vi "RunMeas.vi"(8 "error in (no error)":errorcluster, 11 "NhRegenGridSim in":refnum<class "NHRGridSim.lvclass">) -> (0 "error out":errorcluster, 2 "variant":variant, 3 "NhRegenGridSim out":refnum<class "NHRGridSim.lvclass">)   [LabVIEW 2018, in "AcPwrPlugins.lvlib" / "NHRGridSim.lvclass"]
doc: "This VI acquires data from the instrument and fetches the data from instrument memory into LabVIEW memory."
uses:
  NHRGridSim.lvclass
  C:/Users/ico/Documents/Projects/NistPluggableModules/AcPwr/AcPwrPlugins/AcPwrBaseClass/AcPwrBase.lvclass
  <instrlib>/NH Research 9400 Series/Public/Data/Low Level/Fetch (Ave Current).vi
  <instrlib>/NH Research 9400 Series/Public/Data/Read (Ave Current).vi
  <instrlib>/NH Research 9400 Series/Public/Data/Low Level/Fetch (Max Current).vi
  <instrlib>/NH Research 9400 Series/Public/Data/Read (Max Current).vi
  <instrlib>/NH Research 9400 Series/Public/Data/Low Level/Fetch (Min Current).vi
  <instrlib>/NH Research 9400 Series/Public/Data/Read (Min Current).vi
  <instrlib>/NH Research 9400 Series/Public/Data/Low Level/Fetch (Ave Voltage).vi
  <instrlib>/NH Research 9400 Series/Public/Data/Read (Ave Voltage).vi
  <instrlib>/NH Research 9400 Series/Public/Data/Low Level/Fetch (Max Voltage).vi
  <instrlib>/NH Research 9400 Series/Public/Data/Read (Max Voltage).vi
  <instrlib>/NH Research 9400 Series/Public/Data/Low Level/Fetch (Min Voltage).vi
  <instrlib>/NH Research 9400 Series/Public/Data/Read (Min Voltage).vi
  <instrlib>/NH Research 9400 Series/Public/Data/Low Level/Fetch (Ave True Power).vi
  <instrlib>/NH Research 9400 Series/Public/Data/Read (Ave True Power).vi
  <instrlib>/NH Research 9400 Series/Public/Data/Low Level/Fetch (Max True Power).vi
  <instrlib>/NH Research 9400 Series/Public/Data/Read (Max True Power).vi
  <instrlib>/NH Research 9400 Series/Public/Data/Low Level/Fetch (Min True Power).vi
  <instrlib>/NH Research 9400 Series/Public/Data/Read (Min True Power).vi
  <instrlib>/NH Research 9400 Series/Public/Data/Low Level/Fetch (Ave Apparent Power).vi
  <instrlib>/NH Research 9400 Series/Public/Data/Read (Ave Apparent Power).vi
  <instrlib>/NH Research 9400 Series/Public/Data/Low Level/Fetch (Max Apparent Power).vi
  <instrlib>/NH Research 9400 Series/Public/Data/Read (Max Apparent Power).vi
  <instrlib>/NH Research 9400 Series/Public/Data/Low Level/Fetch (Min Apparent Power).vi
  <instrlib>/NH Research 9400 Series/Public/Data/Read (Min Apparent Power).vi
  <instrlib>/NH Research 9400 Series/Public/Data/Low Level/Fetch (Power Factor).vi
  <instrlib>/NH Research 9400 Series/Public/Data/Read (Power Factor).vi
  <instrlib>/NH Research 9400 Series/Public/Data/Low Level/Fetch (Crest Factor).vi
  <instrlib>/NH Research 9400 Series/Public/Data/Read (Crest Factor).vi
  <instrlib>/NH Research 9400 Series/NH Research 9400 Series.lvlib
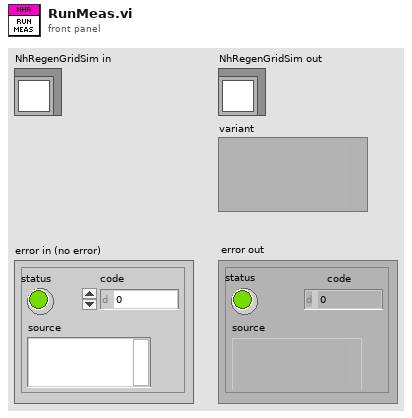
[diagram p1: front panel]
types:
  T1 = typedef "AcPwrPlugins.lvlib/NhRegenGridSim.lvclass/Measurements.ctl" = cluster{"Handle":string, "Name":string, "Enabled ":bool, "Measurement Value":dbl, "Measurement Type ":enum16{"Average Current", "Max Current", "Min Current", "Average Voltage", "Max Voltage", "Min Voltage", "Average True Power", "Max True Power", "Min True Power", "Average Apparent Power", "Max Apparent Power", "Min Apparent Power", "Power Factor", "Crest Factor"}, "Phase ":i32, "btnMeasFetch":bool}[]
  T2 = enum16{"Average Current", "Max Current", "Min Current", "Average Voltage", "Max Voltage", "Min Voltage", "Average True Power", "Max True Power", "Min True Power", "Average Apparent Power", "Max Apparent Power", "Min Apparent Power", "Power Factor", "Crest Factor"}
  T3 = cluster{"Handle":string, "Name":string, "Enabled ":bool, "Measurement Value":dbl, "Measurement Type ":enum16{"Average Current", "Max Current", "Min Current", "Average Voltage", "Max Voltage", "Min Voltage", "Average True Power", "Max True Power", "Min True Power", "Average Apparent Power", "Max Apparent Power", "Min Apparent Power", "Power Factor", "Crest Factor"}, "Phase ":i32, "btnMeasFetch":bool}
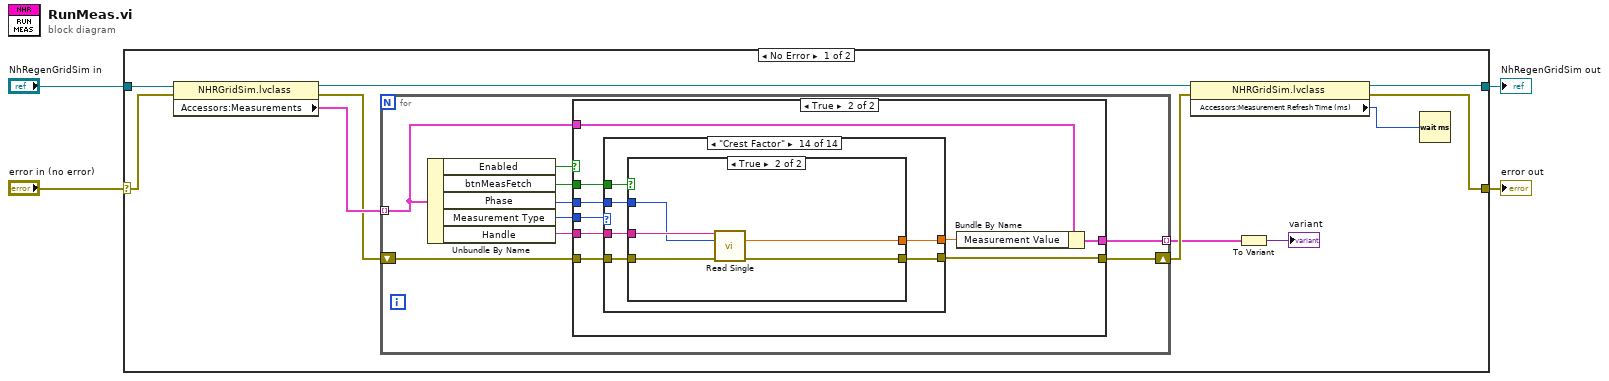
[diagram p0: block diagram]
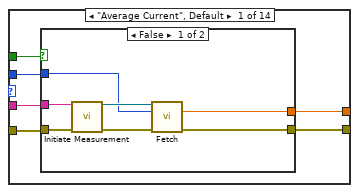
[diagram p3: hidden frame]
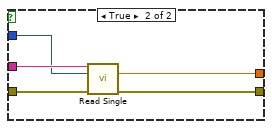
[diagram p4: hidden frame]
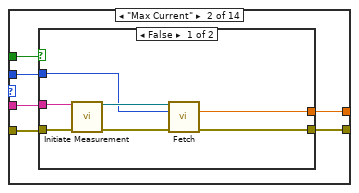
[diagram p5: hidden frame]
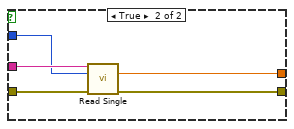
[diagram p6: hidden frame]
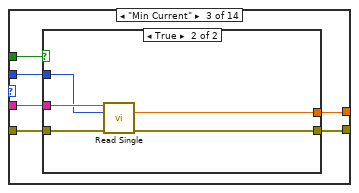
[diagram p7: hidden frame]
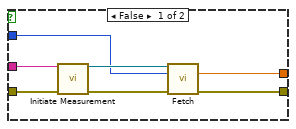
[diagram p8: hidden frame]
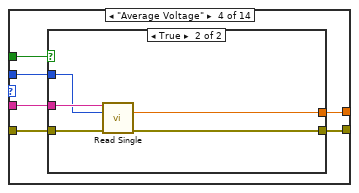
[diagram p9: hidden frame]
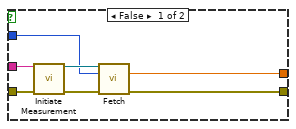
[diagram p10: hidden frame]
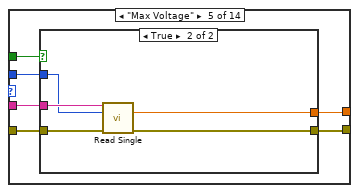
[diagram p11: hidden frame]
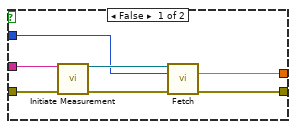
[diagram p12: hidden frame]
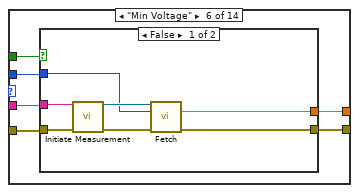
[diagram p13: hidden frame]
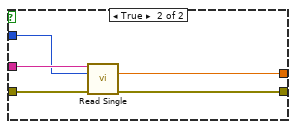
[diagram p14: hidden frame]
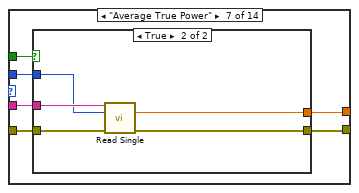
[diagram p15: hidden frame]
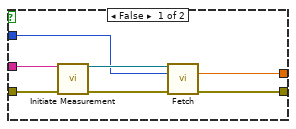
[diagram p16: hidden frame]
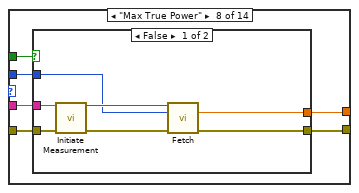
[diagram p17: hidden frame]
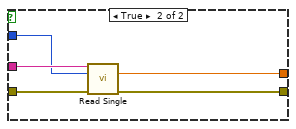
[diagram p18: hidden frame]
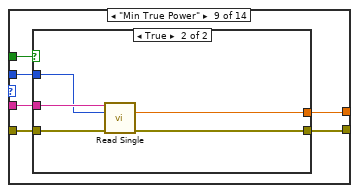
[diagram p19: hidden frame]
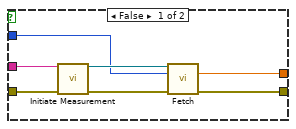
[diagram p20: hidden frame]
diagram:
  n1 = case shown="No Error" "error in (no error)" {
    selector: "error in (no error)" -> [w14 w287]
    tunnel: [w8 w287] -> w4
    tunnel: [w9 w288] -> w3
    tunnel: "NhRegenGridSim in" -> [w15 w288]
    frame No Error {
      n2 = property class="NHRGridSim.lvclass"(reference=w15, error in=w14) -> (reference out=w11:refnum<class "NHRGridSim.lvclass">, error out=w12:errorcluster, "Accessors:Measurements"=w13:T1)
      n3 = for {
        tunnel: w13 -> [w24] mode=indexing
        shift-right: [w21] -> w10
        shift-left: w12 -> [w23]
        tunnel: [w18] -> w5 mode=indexing
        n4 = Unbundle By Name(w24) -> ("Enabled"=w16:bool, "btnMeasFetch"=w20:bool, "Phase"=w19:i32, "Measurement Type"=w17:T2, "Handle"=w22:string)
        n5 = case shown="True" w16 {
          tunnel: w24 -> [_ w33]
          tunnel: w23 -> [w25 w30]
          tunnel: w22 -> [_ w29]
          tunnel: [w25 w27] -> w21
          tunnel: w19 -> [_ w31]
          tunnel: [_ w34] -> w18
          tunnel: w17 -> [_ w32]
          tunnel: w20 -> [_ w28]
          frame False {
          }
          frame True {
            n6 = case shown="\"Crest Factor\"" w32 {
              tunnel: w31 -> [w37 w54 w72 w90 w108 w126 w144 w162 w180 w198 w216 w234 w252 w270]
              tunnel: w30 -> [w40 w58 w74 w92 w110 w128 w146 w164 w182 w200 w218 w236 w254 w272]
              tunnel: w29 -> [w38 w55 w73 w91 w109 w127 w145 w163 w181 w199 w217 w235 w253 w271]
              tunnel: w28 -> [w36 w53 w71 w89 w107 w125 w143 w161 w179 w197 w215 w233 w251 w269]
              tunnel: [w39 w57 w76 w94 w112 w130 w148 w166 w184 w202 w220 w238 w256 w274] -> w27
              tunnel: [w35 w56 w75 w93 w111 w129 w147 w165 w183 w201 w219 w237 w255 w273] -> w26
              frame "Average Current", Default {
                n7 = case shown="False" w36 {
                  tunnel: w40 -> [w47 w52]
                  tunnel: w38 -> [w46 w51]
                  tunnel: [w42 w50] -> w39
                  tunnel: [w41 w49] -> w35
                  tunnel: w37 -> [w43 w48]
                  frame False {
                    n8 = call <instrlib>:"Initiate Measurement.vi"("VISA resource name"=w46, "error in (no error)"=w47) -> ("VISA resource name out"=w44:refnum<visa-resource-name>, "error out"=w45:errorcluster)  [unwired: 12 in]
                    n9 = call-poly <instrlib>:"Fetch.vi"("VISA resource name"=w44, "Phase (0: All)"=w43, "error in (no error)"=w45) -> ("Ave Current (A)"=w41:dbl, "error out"=w42:errorcluster)  [unwired: 10 in, 1 out]
                  }
                  frame True {
                    n10 = call-poly <instrlib>:"Read Single.vi"("VISA resource name"=w51, "Phase (0: All)"=w48, "error in (no error)"=w52) -> ("Ave Current (A)"=w49:dbl, "error out"=w50:errorcluster)  [unwired: 10 in, 1 out]
                  }
                }
              }
              frame "Max Current" {
                n11 = case shown="False" w53 {
                  tunnel: w58 -> [w65 w70]
                  tunnel: w55 -> [w64 w69]
                  tunnel: [w60 w68] -> w57
                  tunnel: [w59 w67] -> w56
                  tunnel: w54 -> [w61 w66]
                  frame False {
                    n12 = call <instrlib>:"Initiate Measurement.vi"("VISA resource name"=w64, "error in (no error)"=w65) -> ("VISA resource name out"=w62:refnum<visa-resource-name>, "error out"=w63:errorcluster)  [unwired: 12 in]
                    n13 = call-poly <instrlib>:"Fetch.vi"("VISA resource name"=w62, "Phase (0: All)"=w61, "error in (no error)"=w63) -> ("Max Current (A)"=w59:dbl, "error out"=w60:errorcluster)  [unwired: 10 in, 1 out]
                  }
                  frame True {
                    n14 = call-poly <instrlib>:"Read Single.vi"("VISA resource name"=w69, "Phase (0: All)"=w66, "error in (no error)"=w70) -> ("Max Current (A)"=w67:dbl, "error out"=w68:errorcluster)  [unwired: 10 in, 1 out]
                  }
                }
              }
              frame "Min Current" {
                n15 = case shown="True" w71 {
                  tunnel: w74 -> [w83 w88]
                  tunnel: w73 -> [w82 w87]
                  tunnel: [w78 w86] -> w76
                  tunnel: [w77 w85] -> w75
                  tunnel: w72 -> [w79 w84]
                  frame False {
                    n16 = call <instrlib>:"Initiate Measurement.vi"("VISA resource name"=w82, "error in (no error)"=w83) -> ("VISA resource name out"=w80:refnum<visa-resource-name>, "error out"=w81:errorcluster)  [unwired: 12 in]
                    n17 = call-poly <instrlib>:"Fetch.vi"("VISA resource name"=w80, "Phase (0: All)"=w79, "error in (no error)"=w81) -> ("Min Current (A)"=w77:dbl, "error out"=w78:errorcluster)  [unwired: 10 in, 1 out]
                  }
                  frame True {
                    n18 = call-poly <instrlib>:"Read Single.vi"("VISA resource name"=w87, "Phase (0: All)"=w84, "error in (no error)"=w88) -> ("Min Current (A)"=w85:dbl, "error out"=w86:errorcluster)  [unwired: 10 in, 1 out]
                  }
                }
              }
              frame "Average Voltage" {
                n19 = case shown="True" w89 {
                  tunnel: w92 -> [w101 w106]
                  tunnel: w91 -> [w100 w105]
                  tunnel: [w96 w104] -> w94
                  tunnel: [w95 w103] -> w93
                  tunnel: w90 -> [w97 w102]
                  frame False {
                    n20 = call <instrlib>:"Initiate Measurement.vi"("VISA resource name"=w100, "error in (no error)"=w101) -> ("VISA resource name out"=w98:refnum<visa-resource-name>, "error out"=w99:errorcluster)  [unwired: 12 in]
                    n21 = call-poly <instrlib>:"Fetch.vi"("VISA resource name"=w98, "Phase (0: All)"=w97, "error in (no error)"=w99) -> ("Ave Voltage (V)"=w95:dbl, "error out"=w96:errorcluster)  [unwired: 10 in, 1 out]
                  }
                  frame True {
                    n22 = call-poly <instrlib>:"Read Single.vi"("VISA resource name"=w105, "Phase (0: All)"=w102, "error in (no error)"=w106) -> ("Ave Voltage (V)"=w103:dbl, "error out"=w104:errorcluster)  [unwired: 10 in, 1 out]
                  }
                }
              }
              frame "Max Voltage" {
                n23 = case shown="True" w107 {
                  tunnel: w110 -> [w119 w124]
                  tunnel: w109 -> [w118 w123]
                  tunnel: [w114 w122] -> w112
                  tunnel: [w113 w121] -> w111
                  tunnel: w108 -> [w115 w120]
                  frame False {
                    n24 = call <instrlib>:"Initiate Measurement.vi"("VISA resource name"=w118, "error in (no error)"=w119) -> ("VISA resource name out"=w116:refnum<visa-resource-name>, "error out"=w117:errorcluster)  [unwired: 12 in]
                    n25 = call-poly <instrlib>:"Fetch.vi"("VISA resource name"=w116, "Phase (0: All)"=w115, "error in (no error)"=w117) -> ("Max Voltage (V)"=w113:dbl, "error out"=w114:errorcluster)  [unwired: 10 in, 1 out]
                  }
                  frame True {
                    n26 = call-poly <instrlib>:"Read Single.vi"("VISA resource name"=w123, "Phase (0: All)"=w120, "error in (no error)"=w124) -> ("Max Voltage (V)"=w121:dbl, "error out"=w122:errorcluster)  [unwired: 10 in, 1 out]
                  }
                }
              }
              frame "Min Voltage" {
                n27 = case shown="False" w125 {
                  tunnel: w128 -> [w137 w142]
                  tunnel: w127 -> [w136 w141]
                  tunnel: [w132 w140] -> w130
                  tunnel: [w131 w139] -> w129
                  tunnel: w126 -> [w133 w138]
                  frame False {
                    n28 = call <instrlib>:"Initiate Measurement.vi"("VISA resource name"=w136, "error in (no error)"=w137) -> ("VISA resource name out"=w134:refnum<visa-resource-name>, "error out"=w135:errorcluster)  [unwired: 12 in]
                    n29 = call-poly <instrlib>:"Fetch.vi"("VISA resource name"=w134, "Phase (0: All)"=w133, "error in (no error)"=w135) -> ("Min Voltage (V)"=w131:dbl, "error out"=w132:errorcluster)  [unwired: 10 in, 1 out]
                  }
                  frame True {
                    n30 = call-poly <instrlib>:"Read Single.vi"("VISA resource name"=w141, "Phase (0: All)"=w138, "error in (no error)"=w142) -> ("Min Voltage (V)"=w139:dbl, "error out"=w140:errorcluster)  [unwired: 10 in, 1 out]
                  }
                }
              }
              frame "Average True Power" {
                n31 = case shown="True" w143 {
                  tunnel: w146 -> [w155 w160]
                  tunnel: w145 -> [w154 w159]
                  tunnel: [w150 w158] -> w148
                  tunnel: [w149 w157] -> w147
                  tunnel: w144 -> [w151 w156]
                  frame False {
                    n32 = call <instrlib>:"Initiate Measurement.vi"("VISA resource name"=w154, "error in (no error)"=w155) -> ("VISA resource name out"=w152:refnum<visa-resource-name>, "error out"=w153:errorcluster)  [unwired: 12 in]
                    n33 = call-poly <instrlib>:"Fetch.vi"("VISA resource name"=w152, "Phase (0: All)"=w151, "error in (no error)"=w153) -> ("Ave True Power (W)"=w149:dbl, "error out"=w150:errorcluster)  [unwired: 10 in, 1 out]
                  }
                  frame True {
                    n34 = call-poly <instrlib>:"Read Single.vi"("VISA resource name"=w159, "Phase (0: All)"=w156, "error in (no error)"=w160) -> ("True Power (W)"=w157:dbl, "error out"=w158:errorcluster)  [unwired: 10 in, 1 out]
                  }
                }
              }
              frame "Max True Power" {
                n35 = case shown="False" w161 {
                  tunnel: w164 -> [w173 w178]
                  tunnel: w163 -> [w172 w177]
                  tunnel: [w168 w176] -> w166
                  tunnel: [w167 w175] -> w165
                  tunnel: w162 -> [w169 w174]
                  frame False {
                    n36 = call <instrlib>:"Initiate Measurement.vi"("VISA resource name"=w172, "error in (no error)"=w173) -> ("VISA resource name out"=w170:refnum<visa-resource-name>, "error out"=w171:errorcluster)  [unwired: 12 in]
                    n37 = call-poly <instrlib>:"Fetch.vi"("VISA resource name"=w170, "Phase (0: All)"=w169, "error in (no error)"=w171) -> ("Max True Power (W)"=w167:dbl, "error out"=w168:errorcluster)  [unwired: 10 in, 1 out]
                  }
                  frame True {
                    n38 = call-poly <instrlib>:"Read Single.vi"("VISA resource name"=w177, "Phase (0: All)"=w174, "error in (no error)"=w178) -> ("Max True Power (W)"=w175:dbl, "error out"=w176:errorcluster)  [unwired: 10 in, 1 out]
                  }
                }
              }
              frame "Min True Power" {
                n39 = case shown="True" w179 {
                  tunnel: w182 -> [w191 w196]
                  tunnel: w181 -> [w190 w195]
                  tunnel: [w186 w194] -> w184
                  tunnel: [w185 w193] -> w183
                  tunnel: w180 -> [w187 w192]
                  frame False {
                    n40 = call <instrlib>:"Initiate Measurement.vi"("VISA resource name"=w190, "error in (no error)"=w191) -> ("VISA resource name out"=w188:refnum<visa-resource-name>, "error out"=w189:errorcluster)  [unwired: 12 in]
                    n41 = call-poly <instrlib>:"Fetch.vi"("VISA resource name"=w188, "Phase (0: All)"=w187, "error in (no error)"=w189) -> ("Min True Power (W)"=w185:dbl, "error out"=w186:errorcluster)  [unwired: 10 in, 1 out]
                  }
                  frame True {
                    n42 = call-poly <instrlib>:"Read Single.vi"("VISA resource name"=w195, "Phase (0: All)"=w192, "error in (no error)"=w196) -> ("Min True Power (W)"=w193:dbl, "error out"=w194:errorcluster)  [unwired: 10 in, 1 out]
                  }
                }
              }
              frame "Average Apparent Power" {
                n43 = case shown="False" w197 {
                  tunnel: w200 -> [w209 w214]
                  tunnel: w199 -> [w208 w213]
                  tunnel: [w204 w212] -> w202
                  tunnel: [w203 w211] -> w201
                  tunnel: w198 -> [w205 w210]
                  frame False {
                    n44 = call <instrlib>:"Initiate Measurement.vi"("VISA resource name"=w208, "error in (no error)"=w209) -> ("VISA resource name out"=w206:refnum<visa-resource-name>, "error out"=w207:errorcluster)  [unwired: 12 in]
                    n45 = call-poly <instrlib>:"Fetch.vi"("VISA resource name"=w206, "Phase (0: All)"=w205, "error in (no error)"=w207) -> ("Apparent Power (VA)"=w203:dbl, "error out"=w204:errorcluster)  [unwired: 10 in, 1 out]
                  }
                  frame True {
                    n46 = call-poly <instrlib>:"Read Single.vi"("VISA resource name"=w213, "Phase (0: All)"=w210, "error in (no error)"=w214) -> ("Apparent Power (VA)"=w211:dbl, "error out"=w212:errorcluster)  [unwired: 10 in, 1 out]
                  }
                }
              }
              frame "Max Apparent Power" {
                n47 = case shown="True" w215 {
                  tunnel: w218 -> [w227 w232]
                  tunnel: w217 -> [w226 w231]
                  tunnel: [w222 w230] -> w220
                  tunnel: [w221 w229] -> w219
                  tunnel: w216 -> [w223 w228]
                  frame False {
                    n48 = call <instrlib>:"Initiate Measurement.vi"("VISA resource name"=w226, "error in (no error)"=w227) -> ("VISA resource name out"=w224:refnum<visa-resource-name>, "error out"=w225:errorcluster)  [unwired: 12 in]
                    n49 = call-poly <instrlib>:"Fetch.vi"("VISA resource name"=w224, "Phase (0: All)"=w223, "error in (no error)"=w225) -> ("Max Apparent Power (VA)"=w221:dbl, "error out"=w222:errorcluster)  [unwired: 10 in, 1 out]
                  }
                  frame True {
                    n50 = call-poly <instrlib>:"Read Single.vi"("VISA resource name"=w231, "Phase (0: All)"=w228, "error in (no error)"=w232) -> ("Max Apparent Power (VA)"=w229:dbl, "error out"=w230:errorcluster)  [unwired: 10 in, 1 out]
                  }
                }
              }
              frame "Min Apparent Power" {
                n51 = case shown="False" w233 {
                  tunnel: w236 -> [w245 w250]
                  tunnel: w235 -> [w244 w249]
                  tunnel: [w240 w248] -> w238
                  tunnel: [w239 w247] -> w237
                  tunnel: w234 -> [w241 w246]
                  frame False {
                    n52 = call <instrlib>:"Initiate Measurement.vi"("VISA resource name"=w244, "error in (no error)"=w245) -> ("VISA resource name out"=w242:refnum<visa-resource-name>, "error out"=w243:errorcluster)  [unwired: 12 in]
                    n53 = call-poly <instrlib>:"Fetch.vi"("VISA resource name"=w242, "Phase (0: All)"=w241, "error in (no error)"=w243) -> ("Min Apparent Power (VA)"=w239:dbl, "error out"=w240:errorcluster)  [unwired: 10 in, 1 out]
                  }
                  frame True {
                    n54 = call-poly <instrlib>:"Read Single.vi"("VISA resource name"=w249, "Phase (0: All)"=w246, "error in (no error)"=w250) -> ("Min Apparent Power (VA)"=w247:dbl, "error out"=w248:errorcluster)  [unwired: 10 in, 1 out]
                  }
                }
              }
              frame "Power Factor" {
                n55 = case shown="True" w251 {
                  tunnel: w254 -> [w263 w268]
                  tunnel: w253 -> [w262 w267]
                  tunnel: [w258 w266] -> w256
                  tunnel: [w257 w265] -> w255
                  tunnel: w252 -> [w259 w264]
                  frame False {
                    n56 = call <instrlib>:"Initiate Measurement.vi"("VISA resource name"=w262, "error in (no error)"=w263) -> ("VISA resource name out"=w260:refnum<visa-resource-name>, "error out"=w261:errorcluster)  [unwired: 12 in]
                    n57 = call-poly <instrlib>:"Fetch.vi"("VISA resource name"=w260, "Phase (0: All)"=w259, "error in (no error)"=w261) -> ("Power Factor"=w257:dbl, "error out"=w258:errorcluster)  [unwired: 10 in, 1 out]
                  }
                  frame True {
                    n58 = call-poly <instrlib>:"Read Single.vi"("VISA resource name"=w267, "Phase (0: All)"=w264, "error in (no error)"=w268) -> ("Power Factor"=w265:dbl, "error out"=w266:errorcluster)  [unwired: 10 in, 1 out]
                  }
                }
              }
              frame "Crest Factor" {
                n59 = case shown="True" w269 {
                  tunnel: w272 -> [w281 w286]
                  tunnel: w271 -> [w280 w285]
                  tunnel: [w276 w284] -> w274
                  tunnel: [w275 w283] -> w273
                  tunnel: w270 -> [w277 w282]
                  frame False {
                    n60 = call <instrlib>:"Initiate Measurement.vi"("VISA resource name"=w280, "error in (no error)"=w281) -> ("VISA resource name out"=w278:refnum<visa-resource-name>, "error out"=w279:errorcluster)  [unwired: 12 in]
                    n61 = call-poly <instrlib>:"Fetch.vi"("VISA resource name"=w278, "Phase (0: All)"=w277, "error in (no error)"=w279) -> ("Crest Factor"=w275:dbl, "error out"=w276:errorcluster)  [unwired: 10 in, 1 out]
                  }
                  frame True {
                    n62 = call-poly <instrlib>:"Read Single.vi"("VISA resource name"=w285, "Phase (0: All)"=w282, "error in (no error)"=w286) -> ("Crest Factor"=w283:dbl, "error out"=w284:errorcluster)  [unwired: 10 in, 1 out]
                  }
                }
              }
            }
            n63 = Bundle By Name(cluster=w33, "Measurement Value"=w26) -> (w34:T3)
          }
        }
      }
      n64 = property class="NHRGridSim.lvclass"(reference=w11, error in=w10) -> (reference out=w9:refnum<class "NHRGridSim.lvclass">, error out=w8:errorcluster, "Accessors:Measurement Refresh Time (ms)"=w7:u32)
      n65 = To Variant(anything=w5) -> (Variant=→"variant":variant)
      n66 = Wait (ms)(milliseconds to wait=w7) -> ()  [unwired: 1 out]
    }
    frame Error {
    }
  }
  "NhRegenGridSim out" <- w3
  "error out" <- w4
